vi "CI.vi"(7 "Integration Time (1 PLCs)":dbl=1.0, 8 "error in (no error)":errorcluster, 9 "Auto Integration (0: OFF)":i32(ring) items=["OFF", "ON", "ONCE"], 10 "Measurement Function (0: Voltage)":i32(ring) items=["Voltage", "Current", "Resistance", "Charge"], 11 "VISA resource name":refnum<visa-resource-name>) -> (0 "error out":errorcluster, 3 "VISA resource name out":refnum<visa-resource-name>)   [LabVIEW 2017]
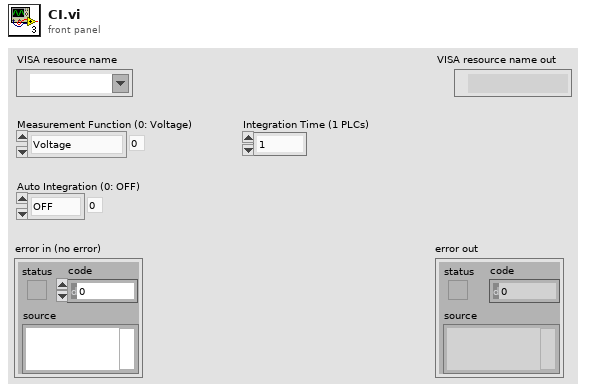
[diagram p1: front panel]
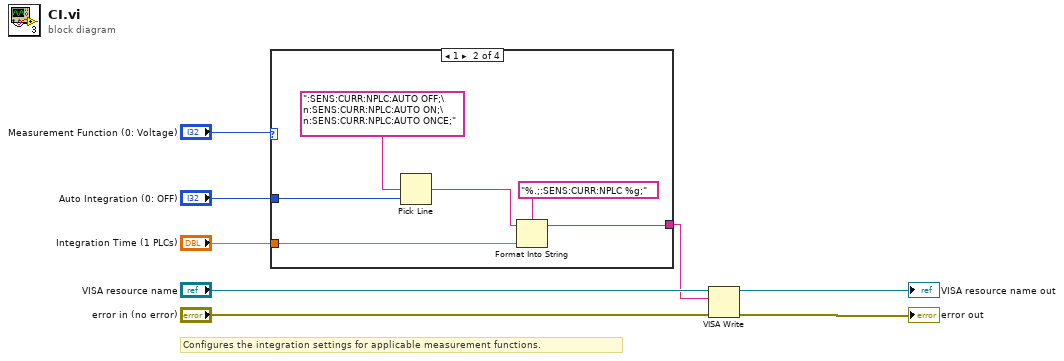
[diagram p0: block diagram]
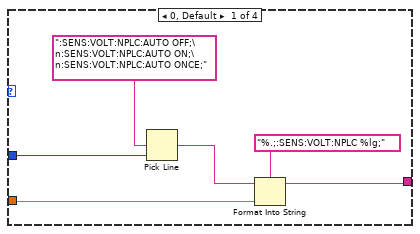
[diagram p2: hidden frame]
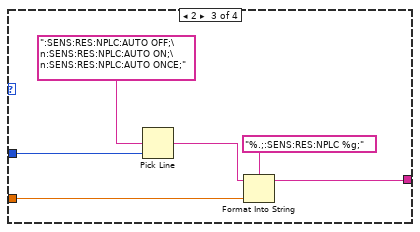
[diagram p3: hidden frame]
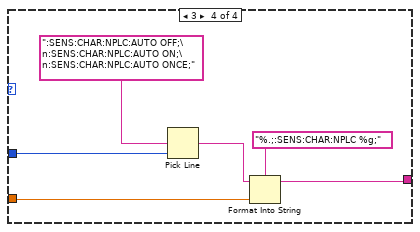
[diagram p4: hidden frame]
diagram:
  # "Configures the integration settings for applicable measurement functions."
  n1 = case shown="1" "Measurement Function (0: Voltage)" {
    tunnel: "Auto Integration (0: OFF)" -> [w13 w19 w25 w29]
    tunnel: "Integration Time (1 PLCs)" -> [w10 w16 w22 w28]
    tunnel: [w9 w15 w21 w27] -> w4
    frame 0, Default {
      n2 = Pick Line(multi-line string=":SENS:VOLT:NPLC:AUTO OFF;\n:SENS:VOLT:NPLC:AUTO ON;\n:SENS:VOLT:NPLC:AUTO ONCE;", line index=w13) -> (output string=w11:string)  [unwired: 1 in]
      n3 = Format Into String(format string="%.;:SENS:VOLT:NPLC %lg;", initial string=w11, w10) -> (resulting string=w9:string)  [unwired: 1 in, 1 out]
    }
    frame 1 {
      n4 = Pick Line(multi-line string=":SENS:CURR:NPLC:AUTO OFF;\n:SENS:CURR:NPLC:AUTO ON;\n:SENS:CURR:NPLC:AUTO ONCE;", line index=w19) -> (output string=w17:string)  [unwired: 1 in]
      n5 = Format Into String(format string="%.;:SENS:CURR:NPLC %g;", initial string=w17, w16) -> (resulting string=w15:string)  [unwired: 1 in, 1 out]
    }
    frame 2 {
      n6 = Pick Line(multi-line string=":SENS:RES:NPLC:AUTO OFF;\n:SENS:RES:NPLC:AUTO ON;\n:SENS:RES:NPLC:AUTO ONCE;", line index=w25) -> (output string=w23:string)  [unwired: 1 in]
      n7 = Format Into String(format string="%.;:SENS:RES:NPLC %g;", initial string=w23, w22) -> (resulting string=w21:string)  [unwired: 1 in, 1 out]
    }
    frame 3 {
      n8 = Pick Line(multi-line string=":SENS:CHAR:NPLC:AUTO OFF;\n:SENS:CHAR:NPLC:AUTO ON;\n:SENS:CHAR:NPLC:AUTO ONCE;", line index=w29) -> (output string=w31:string)  [unwired: 1 in]
      n9 = Format Into String(format string="%.;:SENS:CHAR:NPLC %g;", initial string=w31, w28) -> (resulting string=w27:string)  [unwired: 1 in, 1 out]
    }
  }
  n10 = VISA Write(VISA resource name="VISA resource name", write buffer=w4, error in (no error)="error in (no error)") -> (VISA resource name out=→"VISA resource name out":refnum<visa-resource-name>, error out=→"error out":errorcluster)  [unwired: 1 out]
